vi "flower.vi"() -> ()   [LabVIEW 2022 SP3]
uses:
  <vilib>/Math Plots/3D Math Plots/3D Surface/3D Surface XCtrl/3D Surface.xctl
  <vilib>/Analysis/1siggen.llb/Ramp Pattern by Samples.vi
  <vilib>/gmath/interp.llb/Create Mesh Grid (2D) (x,y arrays).vi
  <vilib>/Math Plots/3D Math Plots/3D Surface/3D Surface Datatype/Public/Plot Helper (Matrix).vi
  <vilib>/Analysis/NI_AALBase.lvlib
  <vilib>/gmath/NI_Gmath.lvlib
  <vilib>/Math Plots/3D Math Plots/3D Surface/3D Surface Datatype/3D Surface Datatype.lvclass
panel:
  out "3D Surface":refnum<class "3D Plot Datatype.lvclass">[](xcontrol)
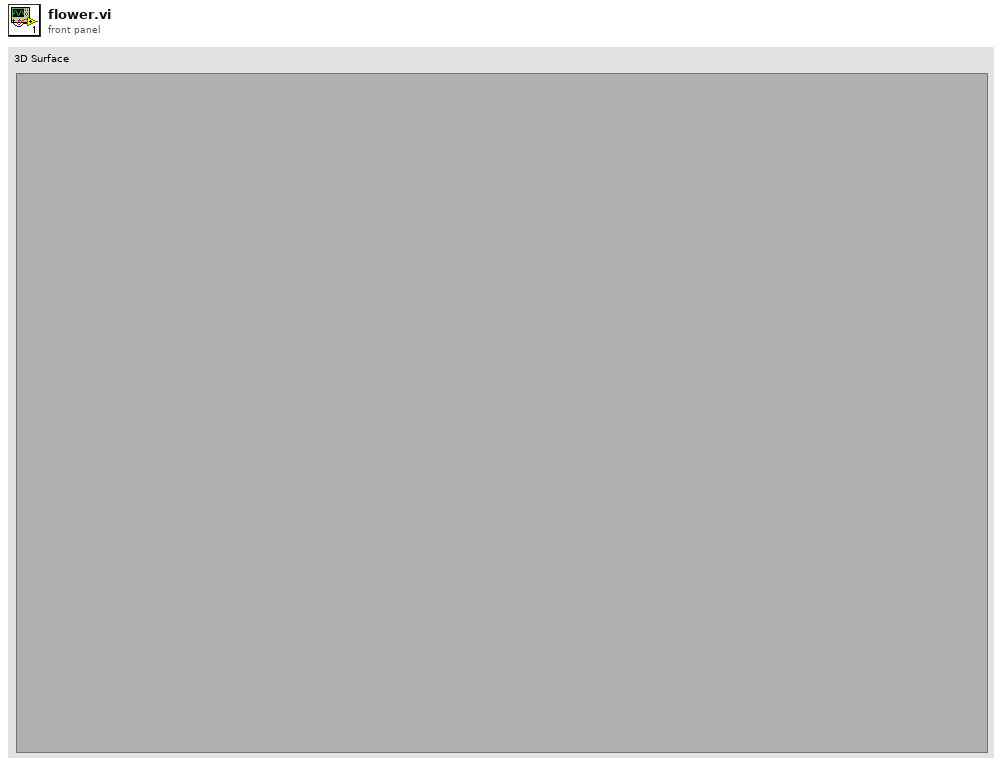
[diagram p1: front panel]
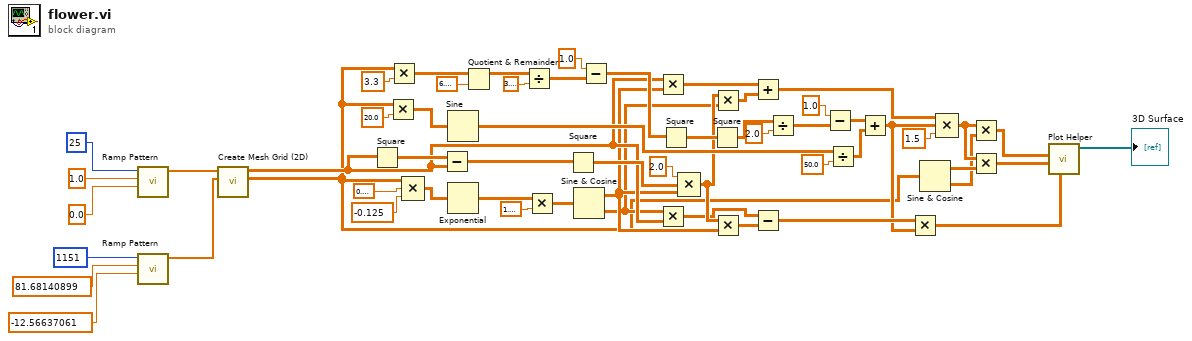
[diagram p0: block diagram]
diagram:
  n1 = call-poly <vilib>:"Ramp Pattern.vi"("start"=0.0, "end"=1.0, "samples"=25) -> ("Ramp Pattern"=w51:dbl[])  [unwired: 7 in, 1 out]
  n2 = call-poly <vilib>:"Ramp Pattern.vi"("start"=-12.56637061, "end"=81.68140899, "samples"=1151) -> ("Ramp Pattern"=w50:dbl[])  [unwired: 7 in, 1 out]
  n3 = call-poly <vilib>:"Create Mesh Grid (2D).vi"("y domain"=w50, "x domain"=w51) -> ("Y"=w3:dbl[][], "X"=w19:dbl[][])  [unwired: 7 in, 1 out]
  n4 = Square(x=w19) -> (x^2=w25:dbl[][])
  n5 = Multiply(x=w3, y=20.0 ("value")) -> (x*y=w43:dbl[][])
  n6 = Multiply(x=w3, y=3.3 ("value")) -> (x*y=w38:dbl[][])
  n7 = Compound Arithmetic op=MULTIPLY(w3, 0.3183098861837907, -0.125 ("value")) -> (w47:dbl[][])
  n8 = Subtract(x=w25, y=w19) -> (x-y=w24:dbl[][])
  n9 = Sine(x=w43) -> (sin(x)=w42:dbl[][])
  n10 = Exponential(1:w47) -> (0:w46:dbl[][])
  n11 = Quotient & Remainder(x=w38, y=6.283185307179586) -> (x-y*floor(x/y)=w37:dbl[][])  [unwired: 1 out]
  n12 = Divide(x=w37, y=3.141592653589793) -> (x/y=w27:dbl[][])
  n13 = Multiply(x=w46, y=1.5707963267948966) -> (x*y=w6:dbl[][])
  n14 = Square(x=w24) -> (x^2=w23:dbl[][])
  n15 = Sine & Cosine(0:w6) -> (1:w5:dbl[][], 2:w4:dbl[][])
  n16 = Subtract(x=1.0, y=w27) -> (x-y=w26:dbl[][])
  n17 = Multiply(x=w19, y=w5) -> (x*y=w21:dbl[][])
  n18 = Multiply(x=w4, y=w19) -> (x*y=w17:dbl[][])
  n19 = Square(x=w26) -> (x^2=w35:dbl[][])
  n20 = Compound Arithmetic op=MULTIPLY(2.0 ("value"), w23, w5) -> (w18:dbl[][])
  n21 = Square(x=w35) -> (x^2=w34:dbl[][])
  n22 = Multiply(x=w18, y=w4) -> (x*y=w20:dbl[][])
  n23 = Multiply(x=w18, y=w5) -> (x*y=w16:dbl[][])
  n24 = Add(x=w21, y=w20) -> (x+y=w15:dbl[][])
  n25 = Subtract(x=w17, y=w16) -> (x-y=w13:dbl[][])
  n26 = Divide(x=w34, y=2.0 ("value")) -> (x/y=w31:dbl[][])
  n27 = Subtract(x=1.0, y=w31) -> (x-y=w30:dbl[][])
  n28 = Divide(x=w42, y=50.0 ("value")) -> (x/y=w29:dbl[][])
  n29 = Add(x=w30, y=w29) -> (x+y=w12:dbl[][])
  n30 = Multiply(x=w13, y=w12) -> (x*y=w8:dbl[][])
  n31 = Sine & Cosine(0:w3) -> (1:w2:dbl[][], 2:w1:dbl[][])
  n32 = Compound Arithmetic op=MULTIPLY(w15, w12, 1.5 ("x")) -> (w10:dbl[][])
  n33 = Multiply(x=w10, y=w1) -> (x*y=w11:dbl[][])
  n34 = Multiply(x=w10, y=w2) -> (x*y=w9:dbl[][])
  n35 = call-poly <vilib>:"Plot Helper.vi"("z matrix"=w8, "y matrix"=w9, "x matrix"=w11) -> ("3D Plot lvclass Array out"=→"3D Surface":refnum<class "3D Plot Datatype.lvclass">[])  [unwired: 3 in, 5 out]
